vi "Folder_creation_calibration.vi"() -> (2 "path":path, 3 "date/time string":string, 4 "calibration log":path)   [LabVIEW 2015]
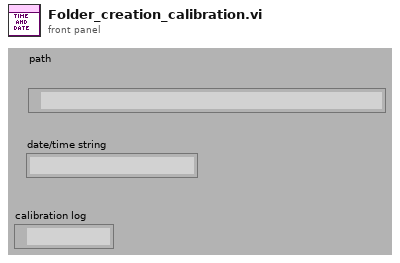
[diagram p1: front panel]
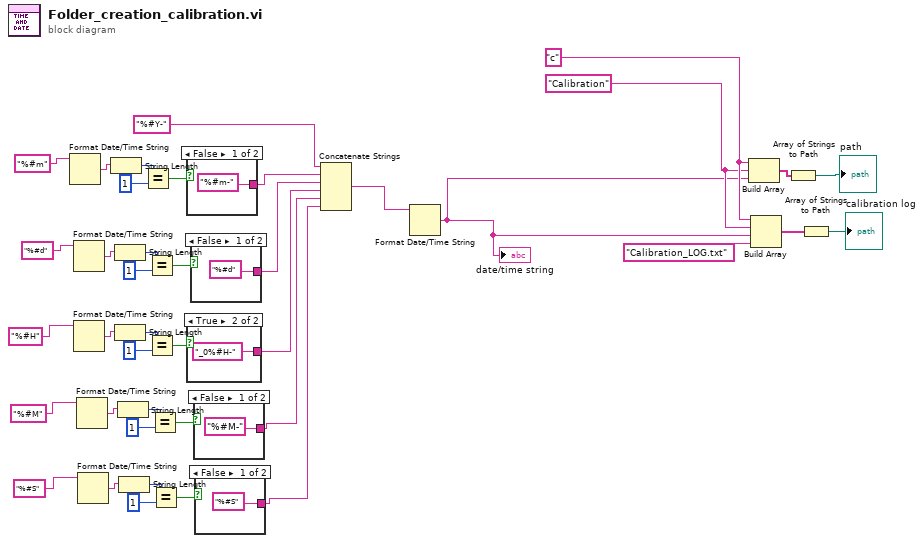
[diagram p0: block diagram]
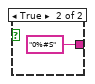
[diagram p2: hidden frame]
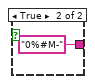
[diagram p3: hidden frame]
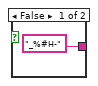
[diagram p4: hidden frame]
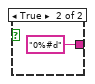
[diagram p5: hidden frame]
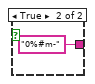
[diagram p6: hidden frame]
diagram:
  w5 = "Calibration" ("element")
  w6 = "c"
  n1 = Format Date/Time String(time format string (%c)="%#m") -> (date/time string=w28:string)  [unwired: 2 in]
  n2 = Format Date/Time String(time format string (%c)="%#d") -> (date/time string=w33:string)  [unwired: 2 in]
  n3 = Format Date/Time String(time format string (%c)="%#H") -> (date/time string=w21:string)  [unwired: 2 in]
  n4 = Format Date/Time String(time format string (%c)="%#M") -> (date/time string=w16:string)  [unwired: 2 in]
  n5 = Format Date/Time String(time format string (%c)="%#S") -> (date/time string=w11:string)  [unwired: 2 in]
  n6 = String Length(string=w28) -> (length=w29:i32)
  n7 = String Length(string=w33) -> (length=w34:i32)
  n8 = String Length(string=w21) -> (length=w22:i32)
  n9 = String Length(string=w16) -> (length=w17:i32)
  n10 = String Length(string=w11) -> (length=w12:i32)
  n11 = Equal?(x=w29, y=1) -> (x = y?=w31:bool)
  n12 = Equal?(x=w34, y=1) -> (x = y?=w36:bool)
  n13 = Equal?(x=w22, y=1) -> (x = y?=w24:bool)
  n14 = Equal?(x=w17, y=1) -> (x = y?=w19:bool)
  n15 = Equal?(x=w12, y=1) -> (x = y?=w14:bool)
  n16 = case shown="False" w31 {
    tunnel: ["%#m-" ("time format string (%c)") "0%#m-" ("time format string (%c)")] -> w38
    frame False {
    }
    frame True {
    }
  }
  n17 = case shown="True" w24 {
    tunnel: ["_%#H-" ("time format string (%c)") "_0%#H-" ("time format string (%c)")] -> w9
    frame False {
    }
    frame True {
    }
  }
  n18 = case shown="False" w36 {
    tunnel: ["%#d" ("time format string (%c)") "0%#d" ("time format string (%c)")] -> w39
    frame False {
    }
    frame True {
    }
  }
  n19 = case shown="False" w19 {
    tunnel: ["%#M-" ("time format string (%c)") "0%#M-" ("time format string (%c)")] -> w8
    frame False {
    }
    frame True {
    }
  }
  n20 = case shown="False" w14 {
    tunnel: ["%#S" ("time format string (%c)") "0%#S" ("time format string (%c)")] -> w7
    frame False {
    }
    frame True {
    }
  }
  n21 = Concatenate Strings("%#Y-" ("time format string (%c)"), w38, w39, w9, w8, w7) -> (w40:string)
  n22 = Format Date/Time String(time format string (%c)=w40) -> (date/time string=w4:string)  [unwired: 2 in]
  "date/time string" <- w4
  n23 = Build Array(w6, w5, w4) -> (w26:string[])
  n24 = Build Array(w6, w5, w4, "Calibration_LOG.txt" ("element")) -> (w2:string[])
  n25 = Array of Strings to Path(0:w26) -> (2:→"path":path)  [unwired: 1 out]
  n26 = Array of Strings to Path(0:w2) -> (2:→"calibration log":path)  [unwired: 1 out]
